vi "Actor Core.vi"(8 "error in":errorcluster, 11 "ImagingExtractor in":refnum<class "ImagingExtractor.lvclass">) -> (0 "error out":errorcluster, 3 "Actor out":refnum<class "Actor.lvclass">)   [LabVIEW 2014, in "ImagingExtractor.lvclass"]
doc: "(<B>Filename</B>: Actor Framework.lvlib:Actor.lvclass:Actor Core.vi)\n\nReceives messages to the actor, reacts to them, and initiates any error handling that may shut the actor down.\n\nDescendant classes may override this VI to append parallel tasks for the actor to complete while it handles messages. Overrides use the Call Parent Method node."
uses:
  ImagingExtractor.lvclass
  <vilib>/ActorFramework/Actor/Actor.lvclass
  <vilib>/ActorFramework/Actor/Actor.lvclass/Actor.ctl
  <vilib>/ActorFramework/Message Enqueuer/Message Enqueuer.lvclass/Message Enqueuer.ctl
  <vilib>/ActorFramework/Message Enqueuer/Init from Existing Queue.vi
  <vilib>/ActorFramework/Message Enqueuer/Message Enqueuer.lvclass
  Framework/Extractor/AbstractExtractor2D/AbstractExtractor2D.lvclass
  Framework/Interfaces/Viewable Actor/Viewable Actor.lvclass
  Framework/Interfaces/Observable Actor/Observable Actor.lvclass
panel:
  out "Stop":bool=TRUE
  # "NOTHING IS HERE"
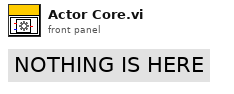
[diagram p1: front panel]
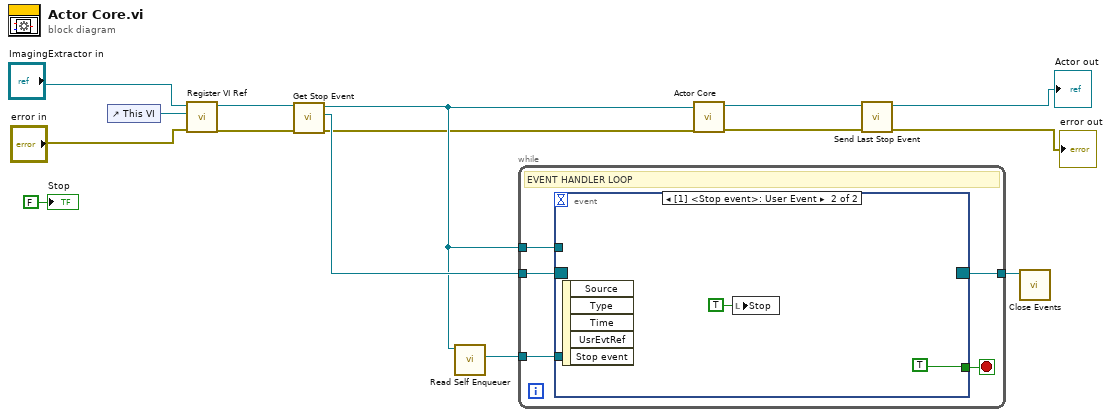
[diagram p0: block diagram]
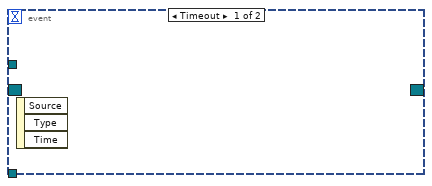
[diagram p2: hidden frame]
diagram:
  n1 = control-ref of="This VI"() -> (w15:refnum<vi>)
  n2 = call "Register VI Ref.vi"("error in (no error)"="error in", "VI ref"=w15, "Viewable Actor in"="ImagingExtractor in") -> ("error out"=w8:errorcluster, "Viewable Actor out"=w9:refnum<class "ImagingExtractor.lvclass">)  [unwired: 7 in]
  n3 = call-dynamic "Get Stop Event.vi"("error in (no error)"=w8, "Observable Actor in"=w9) -> ("error out"=w2:errorcluster, "Events"=w10:refnum<event-registration>, "Observable Actor out"=w3:refnum<class "ImagingExtractor.lvclass">)  [unwired: 7 in]
  n4 = call <vilib>:"Read Self Enqueuer.vi"("Actor"=w3) -> ("Self Enqueuer"=w14:refnum<class "Message Enqueuer.lvclass">)  [unwired: 10 in]
  n5 = while {
    tunnel: w10 -> [w20]
    tunnel: w14 -> [w19]
    tunnel: [w18] -> w11
    tunnel: w3 -> [w16]
    stop <- w17 stop-if-true
    # "EVENT HANDLER LOOP"
    n6 = event shown="[1] <Stop event>: User Event" {
      selector: w20 -> [_ _]
      dyn-events: [_ _] -> w18
      timeout: _ -> [_ _]
      tunnel: w19 -> [_ _]
      tunnel: [_ TRUE] -> w17
      tunnel: w16 -> [_ _]
      event Timeout {
        n7 = event-data() -> ()  [unwired: 1 in, 3 out]
      }
      event User Event {
        n8 = event-data() -> ()  [unwired: 1 in, 5 out]
        n9 = local write "Stop"(TRUE ("Stop")) -> ()
      }
    }
  }
  n10 = call-parent "Actor Core.vi"("error in"=w2, "Actor in"=w3) -> ("error out"=w12:errorcluster, "Actor out"=w13:refnum<class "Actor.lvclass">)  [unwired: 8 in]
  n11 = call "Send Last Stop Event.vi"("error in (no error)"=w12, "Actor in"=w13) -> ("error out"=→"error out":errorcluster, "Actor  out"=→"Actor out":refnum<class "Actor.lvclass">)  [unwired: 8 in]
  n12 = call "Close Events.vi"("events"=w11) -> ()  [unwired: 11 in]
  "Stop" <- FALSE ("Stop")
